vi "_getPropertyValue.vi"   [LabVIEW 2022 SP3, in "openDAQ.lvlib" / "IBaseObject.lvlib" / "IPropertyObject.lvlib" / "IPropertyObject.lvclass"]
uses:
  IPropertyObject.lvclass
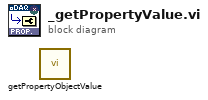
[diagram p0: block diagram]
diagram:
  n1 = call "getPropertyObjectValue.vi"() -> ()  [unwired: 8 in, 4 out]
